vi "Einheiten finden.vi"(10 "Komponente":u16, 11 "Wert":dbl format="%#.6f") -> (0 "Einheit in String":string, 3 "String":string, 4 "Gefunden?":bool, 5 "Wert ppm":dbl, 6 "Komponenten Name":T1)   [LabVIEW 2020, in "Linearisierung v2.lvlib" / "Gasteiler.lvlib"]
uses:
  Gasteiler.lvlib
  Visualisierungs Elemente/String - Ausgabefeld.ctl
  Seiten/Gaszuordnung AO/FGV Gaszuordnung Grenzen&Einheit Aktion.ctl
  Seiten/FT-IR/FGV FT-IR Gasliste Aktionen.ctl
  Aktionen FGV Gasteiler Daten.ctl
  Seiten/Gaszuordnung AO/Gaszuordnung AO.lvlib
  Seiten/FT-IR/FT-IR.lvlib
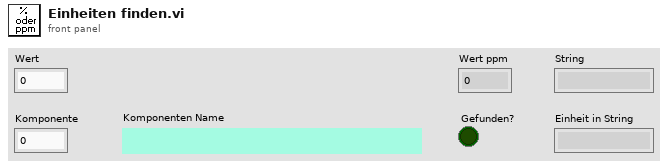
[diagram p1: front panel]
types:
  T1 = typedef "String - Ausgabefeld.ctl" = string
  T2 = typedef "Linearisierung v2.lvlib/Gasteiler.lvlib/Aktionen FGV Gasteiler Daten.ctl" = enum16{"lesen", "Gasteiler Daten", "Seriellen Param.", "MB-Endwert", "laden", "speichern", "Anforderung", "TCP", "Aufzeichnung Start"}
  T3 = typedef "FT-IR.lvlib/FGV FT-IR Gasliste Aktionen.ctl" = enum16{"lesen", "Gasliste FT-IR", "Gasliste ausgelesen", "laden", "speichern", "löschen"}
  T4 = typedef "Gaszuordnung AO.lvlib/FGV Gaszuordnung Grenzen&Einheit Aktion.ctl" = enum16{"Lesen", "Schreiben Min", "Schreiben Max", "Laden", "Speichern"}
  T5 = typedef "Linearisierung v2.lvlib/Gasteiler.lvlib/Gasteiler Daten.ctl" = cluster{"Gasteiler":T6, "Gasteiler Stufen":T7, "Gasteiler Type":T8, "Konfig Gasteiler":T9, "Gasteiler Span Eingänge":u16}
  T6 = typedef "String - Eingabefeld.ctl" = string
  T7 = typedef "Linearisierung v2.lvlib/Gasteiler.lvlib/Gasteiler Stufen.ctl" = u16
  T8 = typedef "Linearisierung v2.lvlib/GasteilerType.ctl" = u16
  T9 = typedef "System Einstellungen V2.lvlib/Gasteiler Auswahl.ctl" = u16
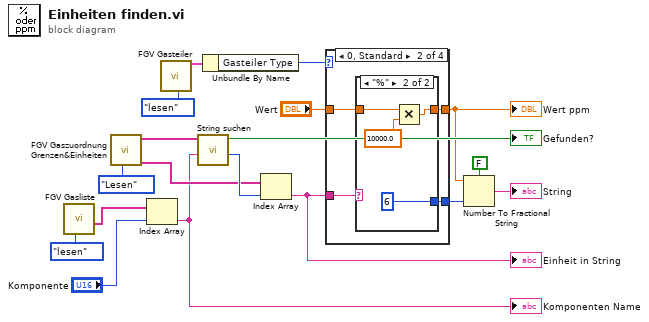
[diagram p0: block diagram]
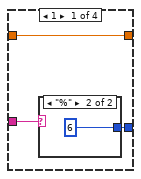
[diagram p2: hidden frame]
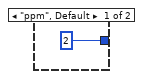
[diagram p3: hidden frame]
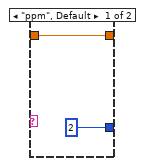
[diagram p4: hidden frame]
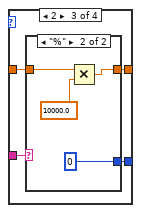
[diagram p5: hidden frame]
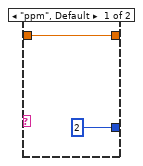
[diagram p6: hidden frame]
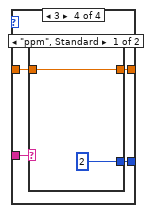
[diagram p7: hidden frame]
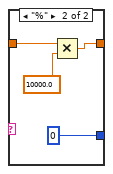
[diagram p8: hidden frame]
diagram:
  n1 = call "FGV Gasliste.vi"("Aktionen"=FGV_FT-IR_Gasliste_Aktionen."lesen") -> ("Aktuelle Gasliste gesamt"=w1:T1[])  [unwired: 8 in, 2 out]
  n2 = call "FGV Gaszuordnung Grenzen&Einheiten.vi"("Aktion"=FGV_Gaszuordnung_Grenzen&Einheit_Aktion."Lesen") -> ("Einheit neu"=w13:string[], "Namen neu"=w9:string[])  [unwired: 7 in, 2 out]
  n3 = Index Array(array=w1, index="Komponente") -> (element=w7:T1)
  "Komponenten Name" <- w7
  n4 = call "FGV Gasteiler.vi"("Aktionen"=Aktionen_FGV_Gasteiler_Daten."lesen") -> ("Gasteiler Daten"=w5:T5)  [unwired: 11 in, 7 out]
  n5 = call "String suchen.vi"("Gasname"=w7, "Such-Namen"=w9) -> ("Index"=w14:i32, "Gefunden?"=→"Gefunden?":bool)  [unwired: 8 in]
  n6 = Unbundle By Name(w5) -> ("Gasteiler Type"=w2:T8)
  n7 = Index Array(array=w13, index=w14) -> (element=w15:string)
  "Einheit in String" <- w15
  n8 = case shown="0, Standard" w2 {
    tunnel: [w21 w27 w37 w47] -> w17
    tunnel: w15 -> [w20 w26 w36 w46]
    tunnel: "Wert" -> [w19 w25 w35 w45]
    tunnel: [w19 w24 w34 w44] -> w3
    frame 1 {
      n9 = case shown="\"%\"" w20 {
        tunnel: [i16 2 ("Genauigkeit (6)") i16 6 ("Genauigkeit (6)")] -> w21
        frame "ppm", Default {
        }
        frame "%" {
        }
      }
    }
    frame 0, Default {
      n10 = case shown="\"%\"" w26 {
        tunnel: [i16 2 ("Genauigkeit (6)") i16 6 ("Genauigkeit (6)")] -> w27
        tunnel: w25 -> [w28 w32]
        tunnel: [w28 w31] -> w24
        frame "ppm", Default {
        }
        frame "%" {
          n11 = Multiply(x=w32, y=sgl 10000.0) -> (x*y=w31:dbl)
        }
      }
    }
    frame 2 {
      n12 = case shown="\"%\"" w36 {
        tunnel: [i16 2 ("Genauigkeit (6)") i16 0 ("Genauigkeit (6)")] -> w37
        tunnel: w35 -> [w38 w42]
        tunnel: [w38 w41] -> w34
        frame "ppm", Default {
        }
        frame "%" {
          n13 = Multiply(x=w42, y=sgl 10000.0) -> (x*y=w41:dbl)
        }
      }
    }
    frame 3 {
      n14 = case shown="\"ppm\", Standard" w46 {
        tunnel: [i16 2 ("Genauigkeit (6)") i16 0 ("Genauigkeit (6)")] -> w47
        tunnel: w45 -> [w48 w52]
        tunnel: [w48 w51] -> w44
        frame "ppm", Default {
        }
        frame "%" {
          n15 = Multiply(x=w52, y=sgl 10000.0) -> (x*y=w51:dbl)
        }
      }
    }
  }
  "Wert ppm" <- w3
  n16 = Number To Fractional String(use system decimal point (T)=FALSE ("Systemdezimalzeichen verwenden (T)"), number=w3, precision (6)=w17) -> (F-format string=→"String":string)  [unwired: 1 in]
